vi "WriteToFile-v2.vi"(0 "Refnum in":refnum<k34>, 1 "Group Name":string, 2 "IO Names":string[](array[string]), 5 "rt fifo":refnum<k33>, 9 "Write?":bool, 11 "error in (no error)":errorcluster, 12 "ConstNames":string[](array[string]), 13 "ConstValues":dbl[](array[numeric])) -> (4 "Refnum out":refnum<k34>, 10 "Writing to file":bool, 15 "error out":errorcluster)   [LabVIEW 2018]
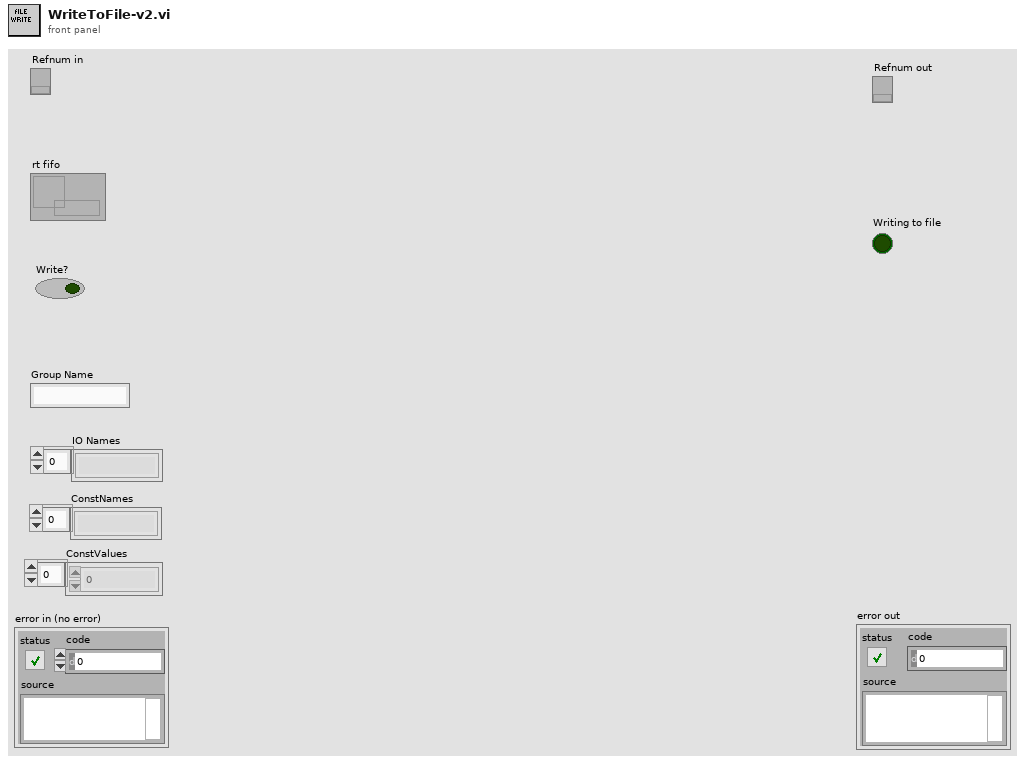
[diagram p1: front panel]
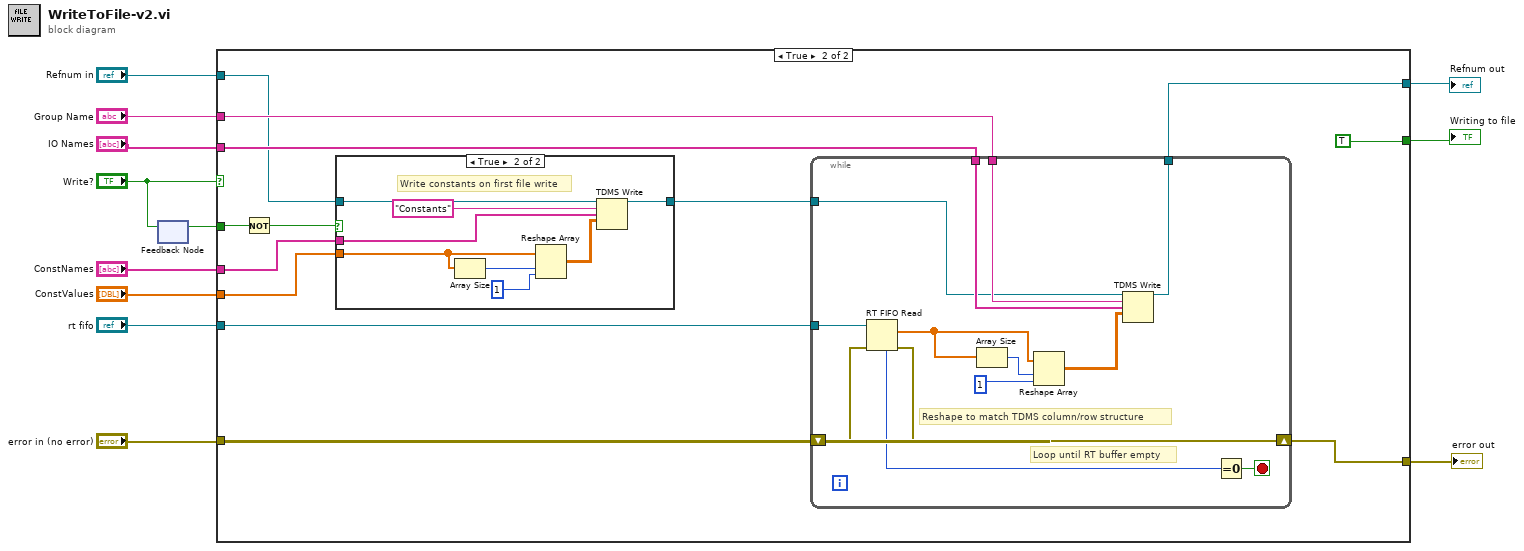
[diagram p0: block diagram]
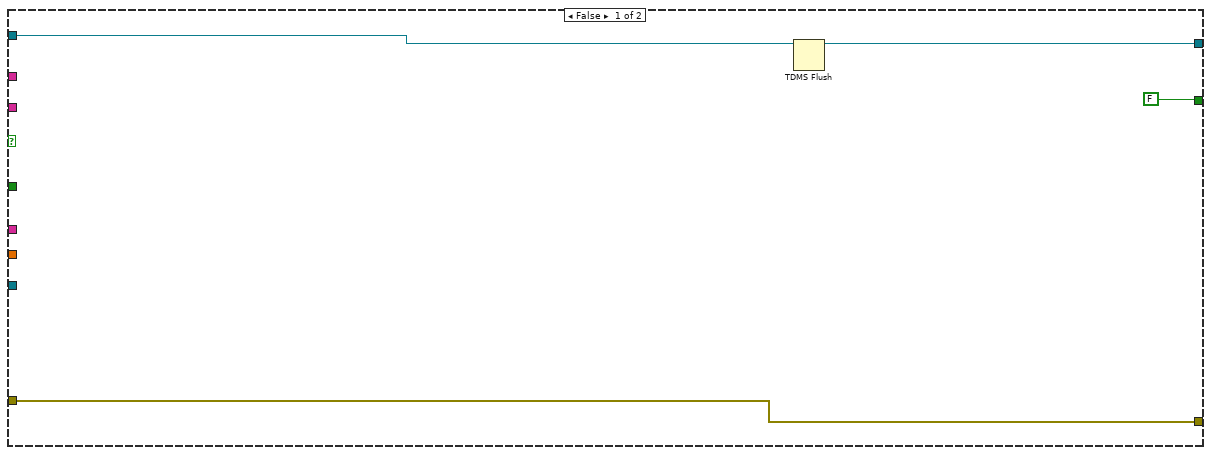
[diagram p2: hidden frame]
diagram:
  n1 = feedback #1() -> (w3:bool)  [unwired: 1 in]
  n2 = feedback-in #1("Write?") -> ()
  n3 = case shown="True" "Write?" {
    tunnel: "Refnum in" -> [w14 w22]
    tunnel: [w13 w24] -> w9
    tunnel: [w15 w23] -> w10
    tunnel: "IO Names" -> [_ w26]
    tunnel: "Group Name" -> [_ w25]
    tunnel: [FALSE ("Writing to file") TRUE ("Writing to file")] -> w7
    tunnel: "rt fifo" -> [_ w27]
    tunnel: "error in (no error)" -> [w15 w28]
    tunnel: w3 -> [_ w20]
    tunnel: "ConstNames" -> [_ w18]
    tunnel: "ConstValues" -> [_ w17]
    frame False {
      n4 = TDMS Flush(7:w14) -> (3:w13:refnum<k34>)  [unwired: 1 in, 1 out]
    }
    frame True {
      n5 = Not(x=w20) -> (.not. x?=w19:bool)
      n6 = case shown="True" w19 {
        tunnel: w22 -> [w30 w38]
        tunnel: [w30 w37] -> w21
        tunnel: w18 -> [_ w33]
        tunnel: w17 -> [_ w32]
        frame False {
        }
        frame True {
          # "Write constants on first file write"
          n7 = Array Size(array=w32) -> (size(s)=w34:i32)
          n8 = Reshape Array(w32, w34, 1) -> (w31:dbl[][])
          n9 = TDMS Write(0:w38, 5:"Constants" ("group name in (Untitled)"), 7:w33, 9:w31) -> (4:w37:refnum<k34>)  [unwired: 2 in, 3 out]
        }
      }
      n10 = while {
        tunnel: w27 -> [w51]
        shift-right: [w49] -> w23
        shift-left: w28 -> [w50]
        tunnel: w26 -> [w46]
        tunnel: w25 -> [w45]
        tunnel: [w44] -> w24
        tunnel: w21 -> [w39]
        stop <- w48 stop-if-true
        # "Reshape to match TDMS column/row structure"
        # "Loop until RT buffer empty"
        n11 = RT FIFO Read(0:w51, 3:w50) -> (7:w47:u32, 9:w40:dbl[], 11:w49:errorcluster)  [unwired: 2 in, 2 out]
        n12 = Array Size(array=w40) -> (size(s)=w43:i32)
        n13 = Reshape Array(w40, w43, 1) -> (w41:dbl[][])
        n14 = TDMS Write(0:w39, 5:w45, 7:w46, 9:w41) -> (4:w44:refnum<k34>)  [unwired: 2 in, 3 out]
        n15 = Equal To 0?(x=w47) -> (x = 0?=w48:bool)
      }
    }
  }
  "error out" <- w10
  "Refnum out" <- w9
  "Writing to file" <- w7
